vi "testMaxFileSize (database).vi"(8 "error in (no error)":errorcluster, 11 "TestCase in":refnum<class "Test Max File Size (SQL).lvclass">) -> (0 "error out":errorcluster, 3 "TestCase out":refnum<class "Test Max File Size (SQL).lvclass">)   [LabVIEW 2019, in "Test Max File Size (SQL).lvclass"]
uses:
  Test Max File Size (SQL).lvclass
  C:/Program Files/National Instruments/LabVIEW 2024/vi.lib/Astemes/LUnit/Test Case.lvclass
  <vilib>/addons/_TSC/TSC Event Logger/Log/Event Level.ctl
  Log Sinks/SQLite Database/SQLite Database.lvclass
  C:/Program Files/National Instruments/LabVIEW 2024/vi.lib/addons/_TSC/TSC Event Logger/Log Sinks/Log Sinks.lvclass
  <vilib>/addons/_TSC/TSC Event Logger/Log/Log.lvclass/Log.ctl
  Log Sinks/SQLite Database/SQLite Database.lvclass/SQLite Database.ctl
  <vilib>/Astemes/LUnit/Test Case.lvclass/Test Case.ctl
  9400858f-8242-4f0f-a3a8-0c5d1ac263e7.vi
  c654d944-6096-4d70-a8f7-bda8229b2ac3.vi
  <vilib>/Astemes/LUnit/Core/LUnit Test Case/Private/Append Fail Result.vi
  <vilib>/Astemes/LUnit/Core/LUnit Test Case/Private/Append Pass Result.vi
  c654d944-6096-4d70-a8f7-bda8229b2ac3.vi/4479f1b4-f4e5-41cd-8a07-3589632eefcf.vi
  <vilib>/Astemes/LUnit/Core/LUnit Test Case/Private/Run In UI.vi
  <vilib>/Utility/error.llb/Clear Errors.vi
  <vilib>/addons/_TSC/TSC Event Logger/Log Sinks/Send Log Packet.vi
  <vilib>/addons/_TSC/TSC Event Logger/TSC Event Logger.lvlib
  <vilib>/addons/_TSC/TSC Event Logger/Log/Log.lvclass
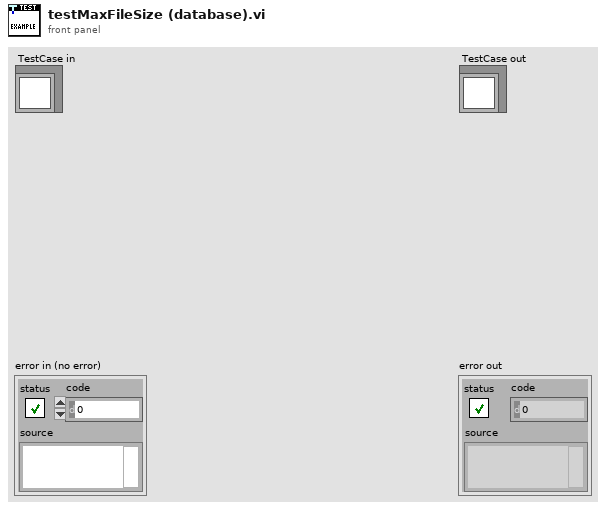
[diagram p1: front panel]
types:
  T1 = typedef "TSC Event Logger.lvlib/Event Level.ctl" = enum16{"OFF", "TRACE", "DEBUG", "INFO", "WARN", "ERROR", "FATAL"}
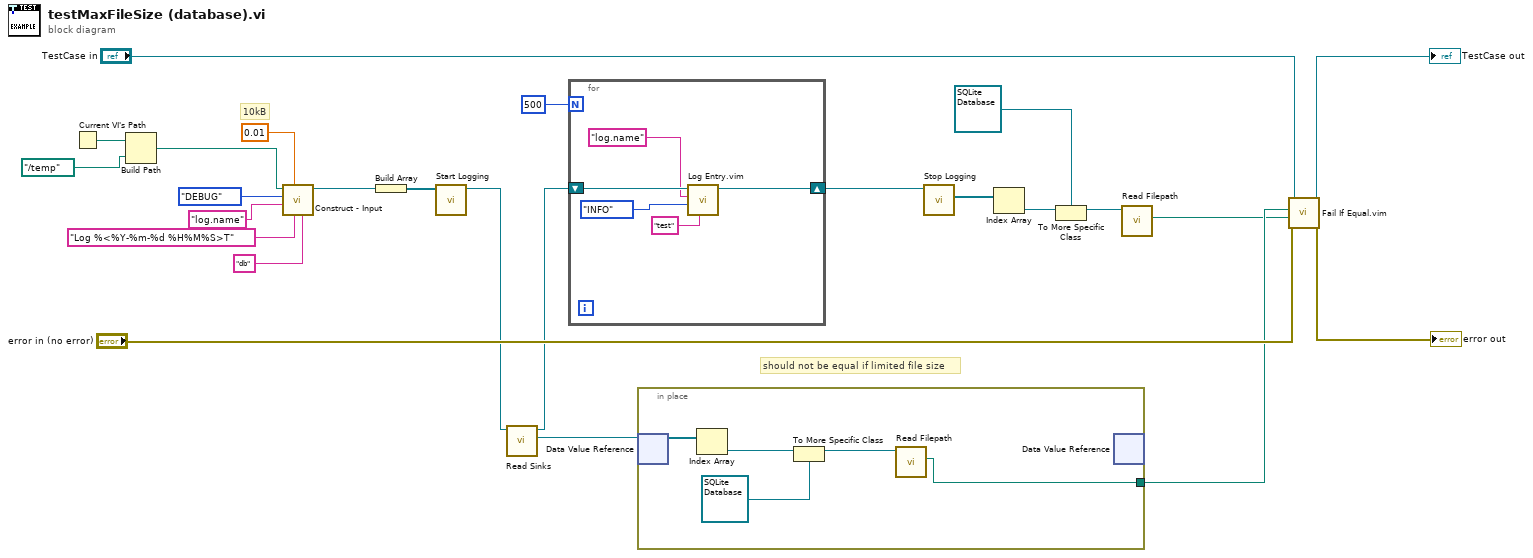
[diagram p0: block diagram]
diagram:
  # "10kB"
  # "should not be equal if limited file size"
  n1 = Current VI's Path() -> (path=w10:path)
  n2 = Build Path(base path=w10, name or relative path=path "../temp") -> (appended path=w12:path)
  n3 = call "Construct - Input.vi"("extension"="db", "file name format"="Log %<%Y-%m-%d %H%M%S>T", "Max File Size (MB)"=0.01, "Name"="log.name", "Level"=Event_Level."DEBUG", "log location"=w12) -> ("SQLite Database out"=w5:refnum<class "SQLite Database.lvclass">)  [unwired: 4 in, 1 out]
  n4 = Build Array(w5) -> (w4:refnum<class "SQLite Database.lvclass">[])
  n5 = call <vilib>:"Start Logging.vi"("Sinks"=w4) -> ("Logger"=w2:refnum<class "Log.lvclass">)  [unwired: 9 in, 1 out]
  n6 = call <vilib>:"Read Sinks.vi"("Log in"=w2) -> ("Sink DVR Array"=w21:refnum<data-value>, "Log out"=w16:refnum<class "Log.lvclass">)  [unwired: 9 in]
  n7 = for {
    N: 500 -> [_]
    shift-right: [w28] -> w17
    shift-left: w16 -> [w29]
    n8 = call "Log Entry.vim"("Message"="test", "Level"=Event_Level."INFO", "Logger"="log.name", "Log in"=w29) -> ("Log out"=w28:refnum<class "Log.lvclass">)  [unwired: 6 in, 1 out]
  }
  n9 = in-place {
    in-place-border: [w31] -> w20
    n10 = in-place-dvr #1(w21) -> (w35:refnum<class "Log Sinks.lvclass">[])  [unwired: 1 out]
    n11 = Index Array(array=w35) -> (element=w34:refnum<class "Log Sinks.lvclass">)  [unwired: 1 in]
    n12 = To More Specific Class(target class=refnum<class "SQLite Database.lvclass"> refnum ("TSC Event Logger (SQL).lvlib:SQLite Database.lvclass"), reference=w34) -> (specific class reference=w33:refnum<class "SQLite Database.lvclass">)  [unwired: 1 in, 1 out]
    n13 = call "Read Filepath.vi"("SQLite Database in"=w33) -> ("File Path Indicator"=w31:path)  [unwired: 9 in, 1 out]
    n14 = in-place-dvr #1() -> ()  [unwired: 1 in, 2 out]
  }
  n15 = call "Stop Logging.vi"("Logger"=w17) -> ("sinks"=w13:refnum<class "Log Sinks.lvclass">[])  [unwired: 9 in, 1 out]
  n16 = Index Array(array=w13) -> (element=w15:refnum<class "Log Sinks.lvclass">)  [unwired: 1 in]
  n17 = To More Specific Class(target class=refnum<class "SQLite Database.lvclass"> refnum ("TSC Event Logger (SQL).lvlib:SQLite Database.lvclass"), reference=w15) -> (specific class reference=w14:refnum<class "SQLite Database.lvclass">)  [unwired: 1 in, 1 out]
  n18 = call "Read Filepath.vi"("SQLite Database in"=w14) -> ("File Path Indicator"=w18:path)  [unwired: 9 in, 1 out]
  n19 = call "Fail If Equal.vim"("error in (no error)"="error in (no error)", "Actual"=w18, "Unexpected"=w20, "LUnit Test Case In"="TestCase in") -> ("error out"=→"error out":errorcluster, "LUnit Test Case Out"=→"TestCase out":refnum<class "Test Max File Size (SQL).lvclass">)  [unwired: 6 in]
